vi "Add Glyph to Icon.vi"() -> ()   [LabVIEW 2023]
uses:
  <vilib>/LabVIEW Icon API/LabVIEW Icon API.lvlib
  <vilib>/LabVIEW Icon API/lv_icon/lv_icon.lvlib
  <vilib>/picture/picture.llb/imagedata.ctl
  <vilib>/Utility/miscctls.llb/LVPoint32TypeDef.ctl
  <vilib>/LabVIEW Icon API/API_User Layer Data.ctl
panel:
  in  "Glyph Path":path
  in  "Control Path":path
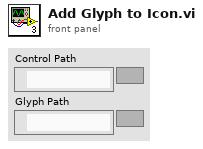
[diagram p1: front panel]
types:
  T1 = typedef "LabVIEW Icon API.lvlib/API_User Layer Data.ctl" = cluster{"Layer name":string, "Origin":T2, "Icon image data":T3}
  T2 = typedef "LVPoint32TypeDef.ctl" = cluster{"Horizontal":i32, "Vertical":i32}
  T3 = typedef "imagedata.ctl" = cluster{"image type":i32, "image depth":i32, "image":u8[], "mask":u8[], "colors":u32[], "Rectangle":cluster{"left":i16, "top":i16, "right":i16, "bottom":i16}}
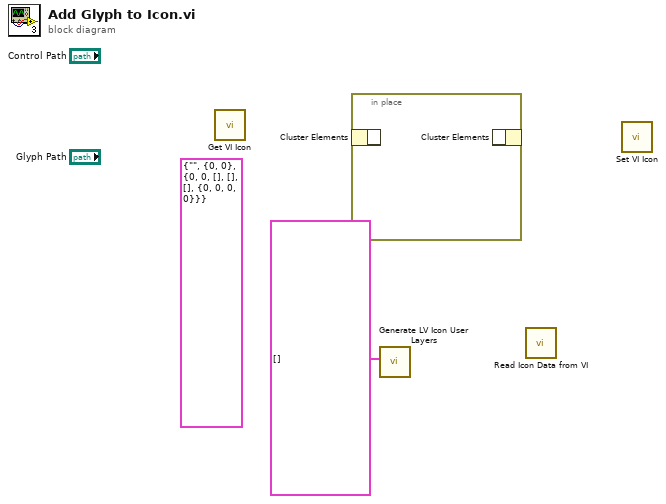
[diagram p0: block diagram]
diagram:
  (unwired) T1 {"Layer name"="", "Origin"={"Horizontal"=0, "Vertical"=0}, "Icon image data"={"image type"=0, "image depth"=0, "image"=[], "mask"=[], "colors"=[], "Rectangle"={"left"=0, "top"=0, "right"=0, "bottom"=0}}} ("User layer")
  n1 = call <vilib>:"Get VI Icon.vi"() -> ()  [unwired: 9 in, 3 out]
  n2 = in-place {
    n3 = in-place-cluster #1() -> ()  [unwired: 1 in, 1 out]
    n4 = in-place-cluster #1() -> ()  [unwired: 1 in, 1 out]
  }
  n5 = call <vilib>:"Generate LV Icon User Layers.vi"("User layers"=T1[] []) -> ()  [unwired: 9 in, 2 out]
  n6 = call <vilib>:"Read Icon Data from VI.vi"() -> ()  [unwired: 9 in, 3 out]
  n7 = call <vilib>:"Set VI Icon.vi"() -> ()  [unwired: 10 in, 2 out]
